vi "Actor Core.vi"(8 "error in":errorcluster, 11 "RandomDataChart in":refnum<class "MultiSubscriber.lvclass">) -> (0 "error out":errorcluster, 3 "Actor out":refnum<class "Actor.lvclass">)   [LabVIEW 2019, in "Integration Test Launcher.lvlib" / "TestViewables.lvlib" / "MultiSubscriber.lvclass"]
doc: "(<B>Filename</B>: Actor Framework.lvlib:Actor.lvclass:Actor Core.vi)\n\nReceives messages to the actor, reacts to them, and initiates any error handling that may shut the actor down.\n\nDescendant classes may override this VI to append parallel tasks for the actor to complete while it handles messages. Overrides use the Call Parent Method node.\n\n<License>\nCopyright © 2020 Tymphany, LLC | All rights reserved\nwww.Tymphany.com\nHuijun <Huijun.Guo@Tymphany.com>\n</License>"
uses:
  <vilib>/gpm_packages/@cs/example/Integration Test/MultiSubscriber/MultiSubscriber.lvclass
  C:/Program Files/National Instruments/LabVIEW 2019/vi.lib/gpm_packages/@cs/mva-viewable/Source/IViewable/IViewable/IViewable.lvclass
  C:/Program Files/National Instruments/LabVIEW 2019/vi.lib/gpm_packages/@cs/mva-core/Source/IObserver/IObserver/IObserver.lvclass
  <vilib>/ActorFramework/Actor/Actor.lvclass
  <vilib>/gpm_packages/@cs/example/Integration Test/MultiSubscriber Messages/Notification Msg/UpdateChart Msg.lvclass
  C:/Program Files/National Instruments/LabVIEW 2019/vi.lib/gpm_packages/@cs/transport/Source/Concrete/ActorMessageTransport/Notification Msg/Notification Msg.lvclass
  <vilib>/gpm_packages/@cs/mva-core/Source/SubscriptionPolicy/BasicSubscription/BasicSubscription.lvclass/BasicSubscription.ctl
  <vilib>/gpm_packages/@cs/example/Integration Test/MultiSubscriber/MultiSubscriber.lvclass/MultiSubscriber.ctl
  <vilib>/ActorFramework/Actor/Actor.lvclass/Actor.ctl
  <vilib>/ActorFramework/Message Enqueuer/Message Enqueuer.lvclass/Message Enqueuer.ctl
  <vilib>/gpm_packages/@cs/transport/Source/Concrete/ActorMessageTransport/ActorMessageTransport.lvclass/ActorMessageTransport.ctl
  <vilib>/gpm_packages/@cs/mva-core/Source/IMediator/SubscriptionRequest/SubscriptionRequest.lvclass/SubscriptionRequest.ctl
  <vilib>/gpm_packages/@cs/mva-core/Source/IObserver/IObserver Messages/Subscribe Msg/Subscribe Msg.lvclass/Subscribe Msg.ctl
  <vilib>/gpm_packages/@cs/mva-core/Source/IMediator/SubscriptionRequest/Pack Subscription Request.vi
  <vilib>/gpm_packages/@cs/mva-core/Source/IObserver/IObserver Messages/Subscribe Msg/Send Subscribe.vi
  <vilib>/ActorFramework/Actor/Read Self Enqueuer.vi
  <vilib>/gpm_packages/@cs/transport/Source/Concrete/ActorMessageTransport/Construct Actor Message Transport.vi
  <vilib>/ActorFramework/Message Enqueuer/Enqueue.vi
  <vilib>/ActorFramework/Message Enqueuer/Init from Existing Queue.vi
  <vilib>/ActorFramework/Message Enqueuer/Equals Not A Refnum.vi
  <vilib>/gpm_packages/@cs/mva-core/Source/SubscriptionPolicy/BasicSubscription/BasicSubscription.lvclass
  C:/Program Files/National Instruments/LabVIEW 2019/vi.lib/gpm_packages/@cs/mva-core/Source/IMediator/ISubscriptionPolicy/ISubscriptionPolicy.lvclass
  <vilib>/gpm_packages/@cs/mva-core/Source/IObserver/IObserver/IObserver.lvclass
  C:/Program Files/National Instruments/LabVIEW 2019/vi.lib/ActorFramework/Actor/Actor.lvclass
  <vilib>/gpm_packages/@cs/transport/Source/Concrete/ActorMessageTransport/ActorMessageTransport.lvclass
  C:/Program Files/National Instruments/LabVIEW 2019/vi.lib/gpm_packages/@cs/transport/Source/ITransport/ITransport.lvclass
  <vilib>/gpm_packages/@cs/mva-core/Source/IObserver/IObserver Messages/Subscribe Msg/Subscribe Msg.lvclass
  C:/Program Files/National Instruments/LabVIEW 2019/vi.lib/ActorFramework/Message/Message.lvclass
  <vilib>/Utility/error.llb/Error Cluster From Error Code.vi
  <vilib>/gpm_packages/@cs/mva-core/Source/IMediator/ISubscriptionPolicy/Open Subscription Policy.vi
  <vilib>/ActorFramework/Message Priority Queue/Priority Enqueue.vi
  <vilib>/ActorFramework/Message Enqueuer/Message Enqueuer.lvclass
  <vilib>/gpm_packages/@cs/mva-core/Source/IMediator/SubscriptionRequest/SubscriptionRequest.lvclass
  <vilib>/gpm_packages/@cs/mva-viewable/Source/IViewable/IViewable/IViewable.lvclass
  <vilib>/gpm_packages/@cs/transport/Source/Concrete/ActorMessageTransport/Notification Msg/Notification Msg.lvclass
panel:
  in  "Process State":dbl
  in  "Launch Dialog":bool
  out "Cluster":T1
  in  "Random Number":dbl
  out "User Value":dbl(graph)
  # "Black Pane\nif Transparency\nis not working\nproperly"
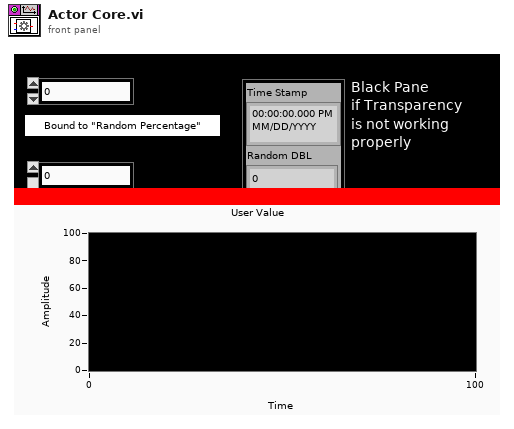
[diagram p1: front panel]
types:
  T1 = cluster{"Time Stamp":timestamp, "Random DBL":dbl}
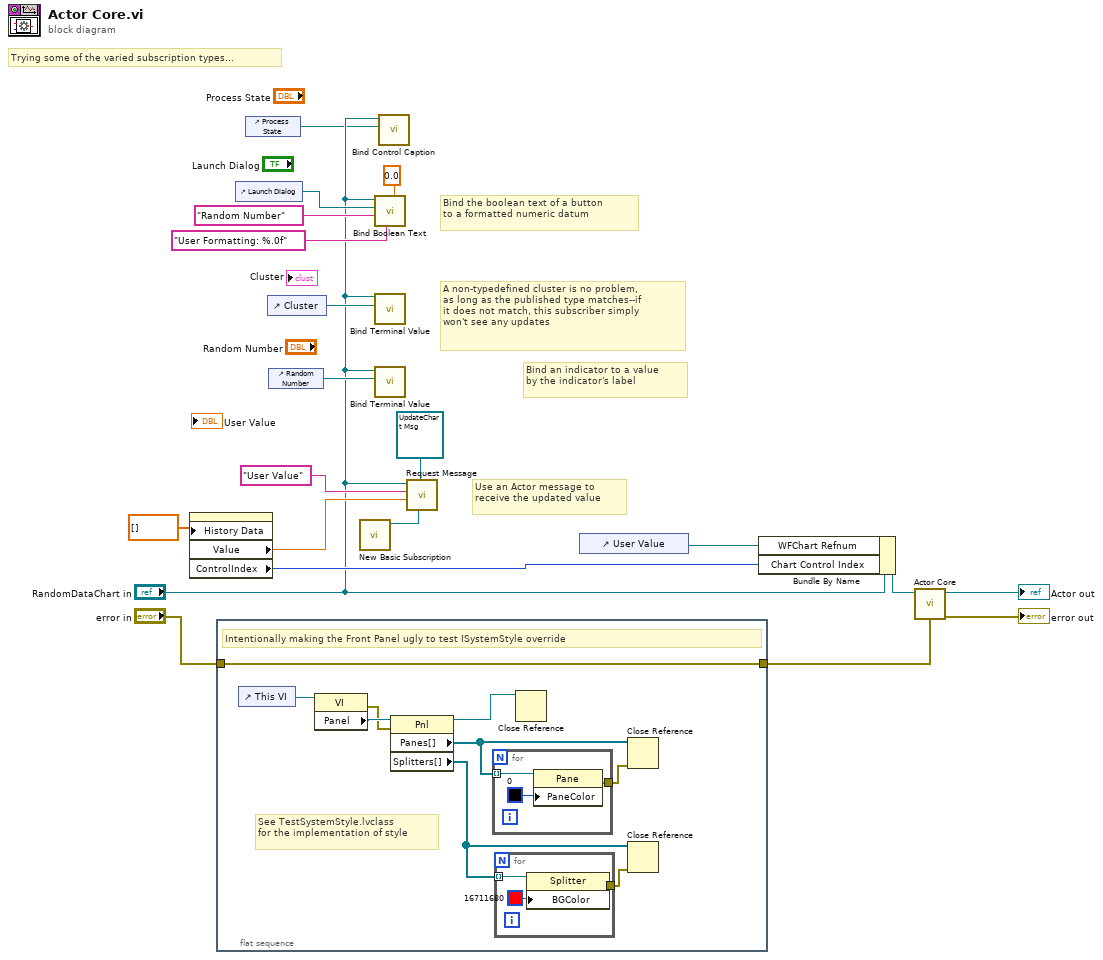
[diagram p0: block diagram]
diagram:
  # "Trying some of the varied subscription types..."
  # "Bind an indicator to a value\nby the indicator's label"
  # "Bind the boolean text of a button\nto a formatted numeric datum"
  # "A non-typedefined cluster is no problem,\nas long as the published type matches--if\nit does not match, this subscriber simply\nwon't see any updates"
  # "Use an Actor message to\nreceive the updated value"
  n1 = property on="User Value" class="WFChart (strict)"("History Data"=dbl[] []) -> ("Value"=w15:dbl, "ControlIndex"=w16:i32)  [unwired: 2 in, 2 out]
  n2 = flat-sequence {
    tunnel: "error in" -> [w23]
    tunnel: [w23] -> w2
    frame #0 {
      # "See TestSystemStyle.lvclass\nfor the implementation of style"
      # "Intentionally making the Front Panel ugly to test ISystemStyle override"
      n3 = control-ref of="This VI"() -> (w29:refnum<vi>)
      n4 = property class="VI"(reference=w29) -> (error out=w21:errorcluster, "Panel"=w28:refnum<vi>)  [unwired: 1 in, 1 out]
      n5 = property class="Pnl"(reference=w28, error in=w21) -> (reference out=w22:refnum<vi>, "Panes[]"=w25:refnum<vi>[], "Splitters[]"=w24:refnum<vi>[])  [unwired: 1 out]
      n6 = for {
        tunnel: [w34] -> w27
        tunnel: w25 -> [w33] mode=indexing
        n7 = property class="Pane"(reference=w33, "PaneColor"=u32 0) -> (error out=w34:errorcluster)  [unwired: 1 in, 1 out]
      }
      n8 = for {
        tunnel: [w31] -> w26
        tunnel: w24 -> [w30] mode=indexing
        n9 = property class="Splitter"(reference=w30, "BGColor"=u32 16711680) -> (error out=w31:errorcluster)  [unwired: 1 in, 1 out]
      }
      n10 = Close Reference(reference=w22) -> ()  [unwired: 1 in, 1 out]
      n11 = Close Reference(reference=w25, error in (no error)=w27) -> ()  [unwired: 1 out]
      n12 = Close Reference(reference=w24, error in (no error)=w26) -> ()  [unwired: 1 out]
    }
  }
  n13 = control-ref of="Launch Dialog"() -> (w6:refnum<vi>)
  n14 = control-ref of="Process State"() -> (w4:refnum<vi>)
  n15 = control-ref of="Cluster"() -> (w7:refnum<vi>)
  n16 = control-ref of="Random Number"() -> (w18:refnum<vi>)
  n17 = call <vilib>:"New Basic Subscription.vi"() -> ("BasicSubscription Out"=w1:refnum<class "BasicSubscription.lvclass">)  [unwired: 11 in]
  n18 = call <vilib>:"Bind Boolean Text.vi"("Datum Type"=0.0, "Format String"="User Formatting: %.0f", "Datum Name (\"\"=Use Control Label)"="Random Number" ("Topic Name (Use Control Text)"), "Bool Refnum"=w6, "IViewable in"="RandomDataChart in") -> ()  [unwired: 5 in, 2 out]
  n19 = call <vilib>:"Bind Terminal Value.vi"("Ctl Refnum"=w7, "IViewable in"="RandomDataChart in") -> ()  [unwired: 8 in, 2 out]
  n20 = call <vilib>:"Bind Terminal Value.vi"("Ctl Refnum"=w18, "IViewable in"="RandomDataChart in") -> ()  [unwired: 8 in, 2 out]
  n21 = call <vilib>:"Bind Control Caption.vi"("Control Refnum"=w4, "IViewable in"="RandomDataChart in") -> ()  [unwired: 8 in, 2 out]
  n22 = call <vilib>:"Request Message.vi"("Configured SubscriptionPolicy"=w1, "Desired Notification Msg"=refnum<class "UpdateChart Msg.lvclass"> refnum ("TestActors.lvlib:MultiSubscriberNotification Msg.lvclass"), "Data Type"=w15, "Datum Name"="User Value" ("Topic Name"), "IObserver in"="RandomDataChart in") -> ()  [unwired: 4 in, 3 out]
  n23 = control-ref of="User Value"() -> (w14:refnum<vi>)
  n24 = Bundle By Name(cluster="RandomDataChart in", "WFChart Refnum"=w14, "Chart Control Index"=w16) -> (w17:refnum<class "MultiSubscriber.lvclass">)
  n25 = call-parent "Actor Core.vi"("error in"=w2, "IViewable In"=w17) -> ("error out"=→"error out":errorcluster, "Actor out"=→"Actor out":refnum<class "Actor.lvclass">)  [unwired: 8 in]
